vi "Write Default Headers.vi"(8 "error in (no error)":errorcluster, 10 "Headers":cluster{"header":string, "value":string}[](array[cluster]), 11 "REST Client_NET in":refnum<class "REST Client_NET.lvclass">) -> (0 "error out":errorcluster, 3 "REST Client_NET out":refnum<class "REST Client_NET.lvclass">)   [LabVIEW 2018, in "REST Client_NET.lvlib" / "REST Client_NET.lvclass"]
doc: "Write Default Headers\n<b> </b> <b> </b>\nHttpClient_NET\nJustin Young - Viviota\nCopyright (c) 2021\nLicense: BSD"
uses:
  REST Client_NET.lvclass
  <vilib>/addons/_JKI.lib/REST Client/classes/REST Client/REST Client.lvclass
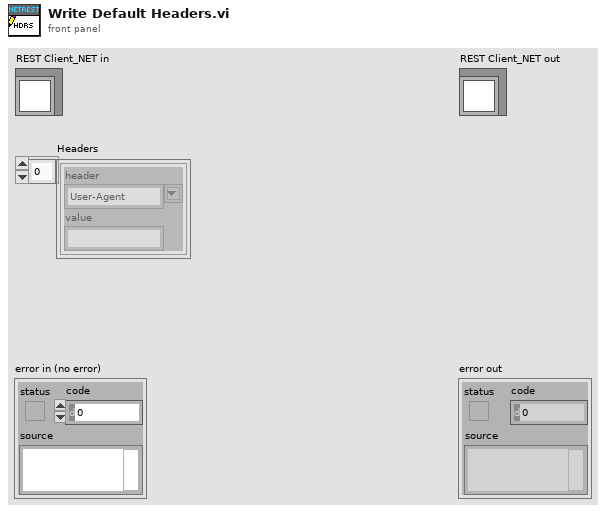
[diagram p1: front panel]
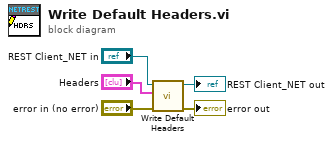
[diagram p0: block diagram]
diagram:
  n1 = call-parent "Write Default Headers.vi"("error in (no error)"="error in (no error)", "Headers"="Headers", "REST Client in"="REST Client_NET in") -> ("error out"=→"error out":errorcluster, "REST Client out"=→"REST Client_NET out":refnum<class "REST Client_NET.lvclass">)  [unwired: 7 in]
